vi "Check Status.vi"(8 "error in (no error)":errorcluster, 11 "Temperature Controller Scientific Instruments in":refnum<class "Temperature Controller Scientific Instruments.lvclass">) -> (0 "error out":errorcluster, 1 "Status":string, 2 "Ready?":bool, 3 "Temperature Controller Scientific Instruments out":refnum<class "Temperature Controller Scientific Instruments.lvclass">)   [LabVIEW 2017, in "Temperature Controller Scientific Instruments.lvclass"]
doc: "(Dynamic) Check if the instrument is powered on and update its member fields with the instrument's current status. Optionally return a text status message."
uses:
  Temperature Controller Scientific Instruments.lvclass
  Utility Classes/Readable/Readable.lvclass
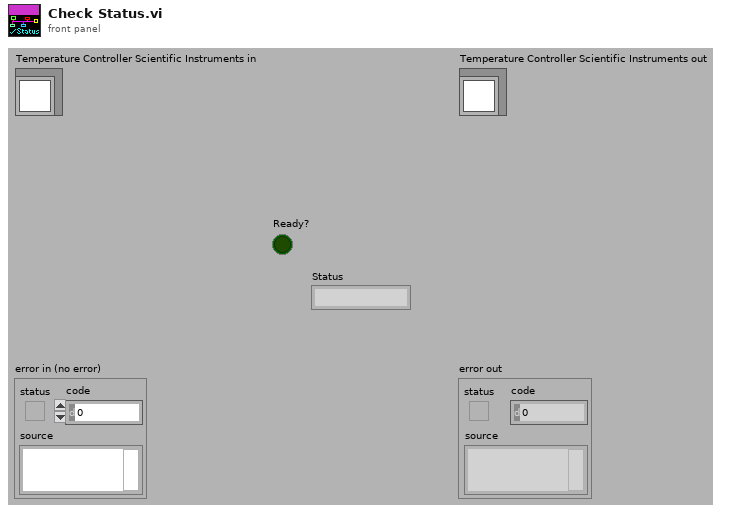
[diagram p1: front panel]
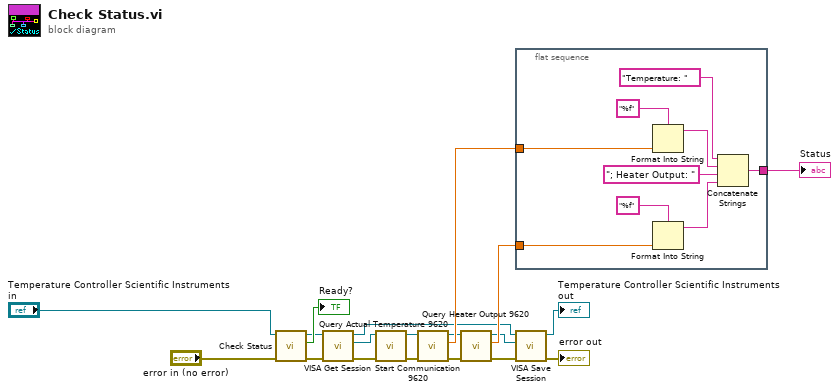
[diagram p0: block diagram]
diagram:
  n1 = call-parent "Check Status.vi"("error in (no error)"="error in (no error)", "Instrument in"="Temperature Controller Scientific Instruments in") -> ("error out"=w5:errorcluster, "Ready?"=→"Ready?":bool, "Instrument out"=w3:refnum<class "Temperature Controller Scientific Instruments.lvclass">)  [unwired: 6 in, 1 out]
  n2 = call-dynamic "VISA Get Session.vi"("error in (no error)"=w5, "Instrument.lvclass in"=w3) -> ("error out"=w6:errorcluster, "VISA Resource Name"=w11:refnum<visa-resource-name>, "Instrument.lvclass out"=w2:refnum<class "Temperature Controller Scientific Instruments.lvclass">)  [unwired: 7 out]
  n3 = call "Start Communication 9620.vi"("error in"=w6, "VISA resource name"=w11) -> ("error out"=w15:errorcluster, "VISA out"=w10:refnum<visa-resource-name>)  [unwired: 8 in]
  n4 = call "Query Actual Temperature 9620.vi"("error in (no error)"=w15, "VISA resource name"=w10) -> ("error out"=w16:errorcluster, "Current actual temperature"=w14:dbl, "VISA resource name out"=w9:refnum<visa-resource-name>)  [unwired: 7 in]
  n5 = call "Query Heater Output 9620.vi"("error in (no error)"=w16, "VISA resource name"=w9) -> ("error out"=w7:errorcluster, "Current heater output"=w13:dbl, "VISA resource name out"=w8:refnum<visa-resource-name>)  [unwired: 7 in]
  n6 = flat-sequence {
    tunnel: [w28] -> w12
    tunnel: w13 -> [w22]
    tunnel: w14 -> [w23]
    frame #0 {
      n7 = Format Into String(format string="%f", w23) -> (resulting string=w21:string)  [unwired: 2 in, 1 out]
      n8 = Format Into String(format string="%f", w22) -> (resulting string=w20:string)  [unwired: 2 in, 1 out]
      n9 = Concatenate Strings("Temperature: " ("string"), w21, "; Heater Output: " ("string"), w20) -> (w28:string)
    }
  }
  n10 = call-dynamic "VISA Save Session.vi"("error in (no error)"=w7, "VISA Resource Name"=w8, "Instrument.lvclass in"=w2) -> ("error out"=→"error out":errorcluster, "Instrument.lvclass out"=→"Temperature Controller Scientific Instruments out":refnum<class "Temperature Controller Scientific Instruments.lvclass">)  [unwired: 7 out]
  "Status" <- w12
